vi "lab5-1.vi"() -> ()   [LabVIEW 2018]
uses:
  <vilib>/DAQmx/configure/timing.llb/DAQmx Timing (Implicit).vi
  <vilib>/DAQmx/create/channels.llb/DAQmx Create Channel (CO-Pulse Generation-Frequency).vi
  <vilib>/DAQmx/create/channels.llb/DAQmx Create Channel (DO-Digital Output).vi
  <vilib>/DAQmx/write.llb/DAQmx Write (Digital Bool 1Line 1Point).vi
panel:
  in  "data":bool=TRUE
  in  "error in 2":errorcluster
  in  "error in":errorcluster
  out "error out":errorcluster
  in  "Frequency":dbl
  in  "samples per channel":i32=1000
  in  "Ring":u16(ring) items=["0", "1"]
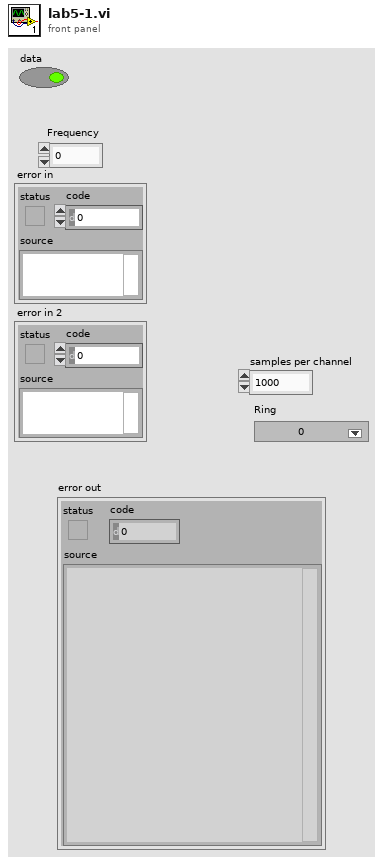
[diagram p1: front panel]
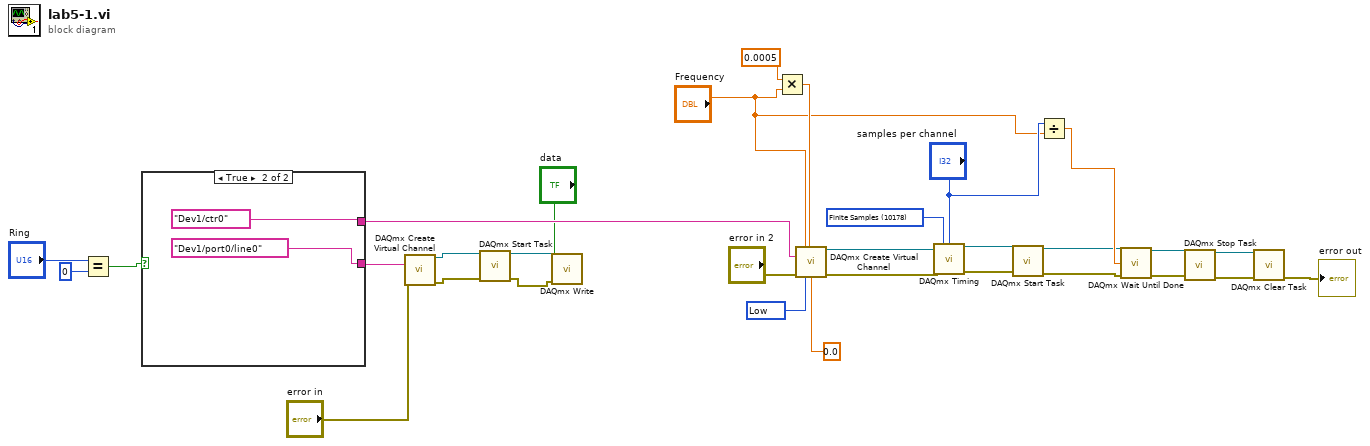
[diagram p0: block diagram]
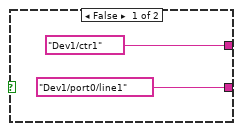
[diagram p2: hidden frame]
diagram:
  w18 = 10214 items=["High"=10192, "Low"=10214] ("idle state")
  w32 = 10178 items=["Finite Samples"=10178, "Continuous Samples"=10123, "Hardware Timed Single Point"=12522] ("sample mode")
  n1 = Equal?(x="Ring", y=u16 0) -> (x = y?=w29:bool)
  n2 = case shown="True" w29 {
    tunnel: [tag "Dev1/ctr1" ("counter") tag "Dev1/ctr0" ("counter")] -> w11
    tunnel: [tag "Dev1/port0/line1" ("lines") tag "Dev1/port0/line0" ("lines")] -> w8
    frame False {
    }
    frame True {
    }
  }
  n3 = call-poly <vilib>:"DAQmx Create Virtual Channel.vi"("lines"=w8, "error in"="error in") -> ("task out"=w7:refnum<k21>, "error out"=w6:errorcluster)  [unwired: 12 in]
  n4 = call <vilib>:"DAQmx Start Task.vi"("task/channels in"=w7, "error in"=w6) -> ("task out"=w4:refnum<k21>, "error out"=w3:errorcluster)  [unwired: 12 in]
  n5 = call-poly <vilib>:"DAQmx Write.vi"("task/channels in"=w4, "data"="data", "error in"=w3) -> ("task out"=w2:refnum<k21>)  [unwired: 10 in, 2 out]
  n6 = Multiply(x=0.0005, y="Frequency") -> (x*y=w27:dbl)
  n7 = call-poly <vilib>:"DAQmx Create Virtual Channel.vi"("frequency"="Frequency", "duty cycle"=w27, "counter"=w11, "error in"="error in 2", "idle state"=w18, "initial delay"=0.0) -> ("task out"=w24:refnum<k21>, "error out"=w25:errorcluster)  [unwired: 8 in]
  n8 = call-poly <vilib>:"DAQmx Timing.vi"("task/channels in"=w24, "sample mode"=w32, "samples per channel"="samples per channel", "error in"=w25) -> ("task out"=w23:refnum<k21>, "error out"=w22:errorcluster)  [unwired: 10 in]
  n9 = call <vilib>:"DAQmx Start Task.vi"("task/channels in"=w23, "error in"=w22) -> ("task out"=w14:refnum<k21>, "error out"=w13:errorcluster)  [unwired: 12 in]
  n10 = Divide(x="samples per channel", y="Frequency") -> (x/y=w15:dbl)
  n11 = call <vilib>:"DAQmx Wait Until Done.vi"("task/channels in"=w14, "timeout (sec)"=w15, "error in"=w13) -> ("task out"=w12:refnum<k21>, "error out"=w1:errorcluster)  [unwired: 11 in]
  n12 = call <vilib>:"DAQmx Stop Task.vi"("task/channels in"=w12, "error in"=w1) -> ("task out"=w21:refnum<k21>, "error out"=w20:errorcluster)  [unwired: 12 in]
  n13 = call <vilib>:"DAQmx Clear Task.vi"("task in"=w21, "error in"=w20) -> ("error out"=→"error out":errorcluster)  [unwired: 13 in]
